vi "4155C Reset.vi"(2 "error in (no error)":errorcluster, 3 "Type of reset":u16(ring) items=["Reset All", "Partial reset"], 4 "VISA session":refnum<visa-resource-name>) -> (0 "error out":errorcluster, 1 "dup VISA resource name":refnum<visa-resource-name>)   [LabVIEW 2019]
doc: "Resets the 4155C with either a hard (false) or soft (true) reset"
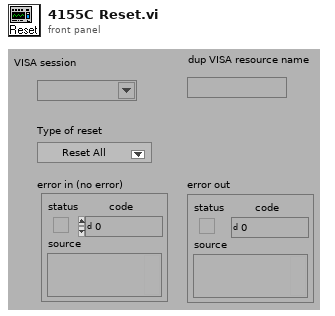
[diagram p1: front panel]
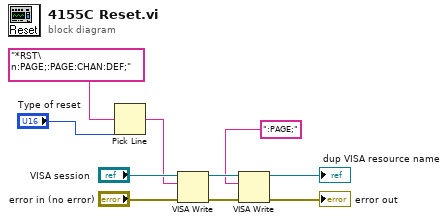
[diagram p0: block diagram]
diagram:
  n1 = Pick Line(multi-line string="*RST\n:PAGE;:PAGE:CHAN:DEF;", line index="Type of reset") -> (output string=w6:string)  [unwired: 1 in]
  n2 = VISA Write(VISA resource name="VISA session", write buffer=w6, error in (no error)="error in (no error)") -> (VISA resource name out=w4:refnum<visa-resource-name>, error out=w5:errorcluster)  [unwired: 1 out]
  n3 = VISA Write(VISA resource name=w4, write buffer=":PAGE;" ("write buffer (\"\")"), error in (no error)=w5) -> (VISA resource name out=→"dup VISA resource name":refnum<visa-resource-name>, error out=→"error out":errorcluster)  [unwired: 1 out]
